vi "Remove Unlogged Channel from Group.vi"(10 "Item Name":string, 11 "References":T1) -> (0 "error out":errorcluster)   [LabVIEW 2015, in "TDMS datalogger editor node.lvclass"]
uses:
  TDMS datalogger editor node.lvclass
  <vilib>/NI/DCAF/Tag Editor Core/Table API/Table Manager/object ref.ctl
  <vilib>/NI/DCAF/Tag Editor Core/Configuration Editor/Classes/Engine Parent/Engine Parent Editor Node.lvclass
  <vilib>/NI/DCAF/Tag Editor Core/Configuration Editor/Classes/Module editor node/module editor node.lvclass
  TDMS datalogger editor node.lvclass/TDMS datalogger editor node.ctl
  <vilib>/NI/DCAF/Tag Editor Core/Table API/Table Manager/Table Manager.lvclass
panel:
  in  "Groups":string(tree)="group1"
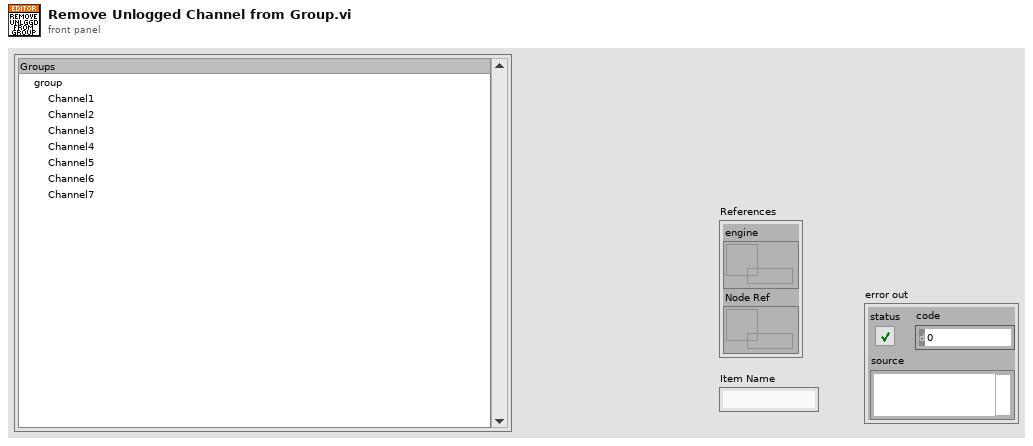
[diagram p1: front panel]
types:
  T1 = typedef "Table Manager.lvlib/Table Manager.lvclass/object ref.ctl" = cluster{"engine":refnum<data-value>, "Node Ref":refnum<data-value>}
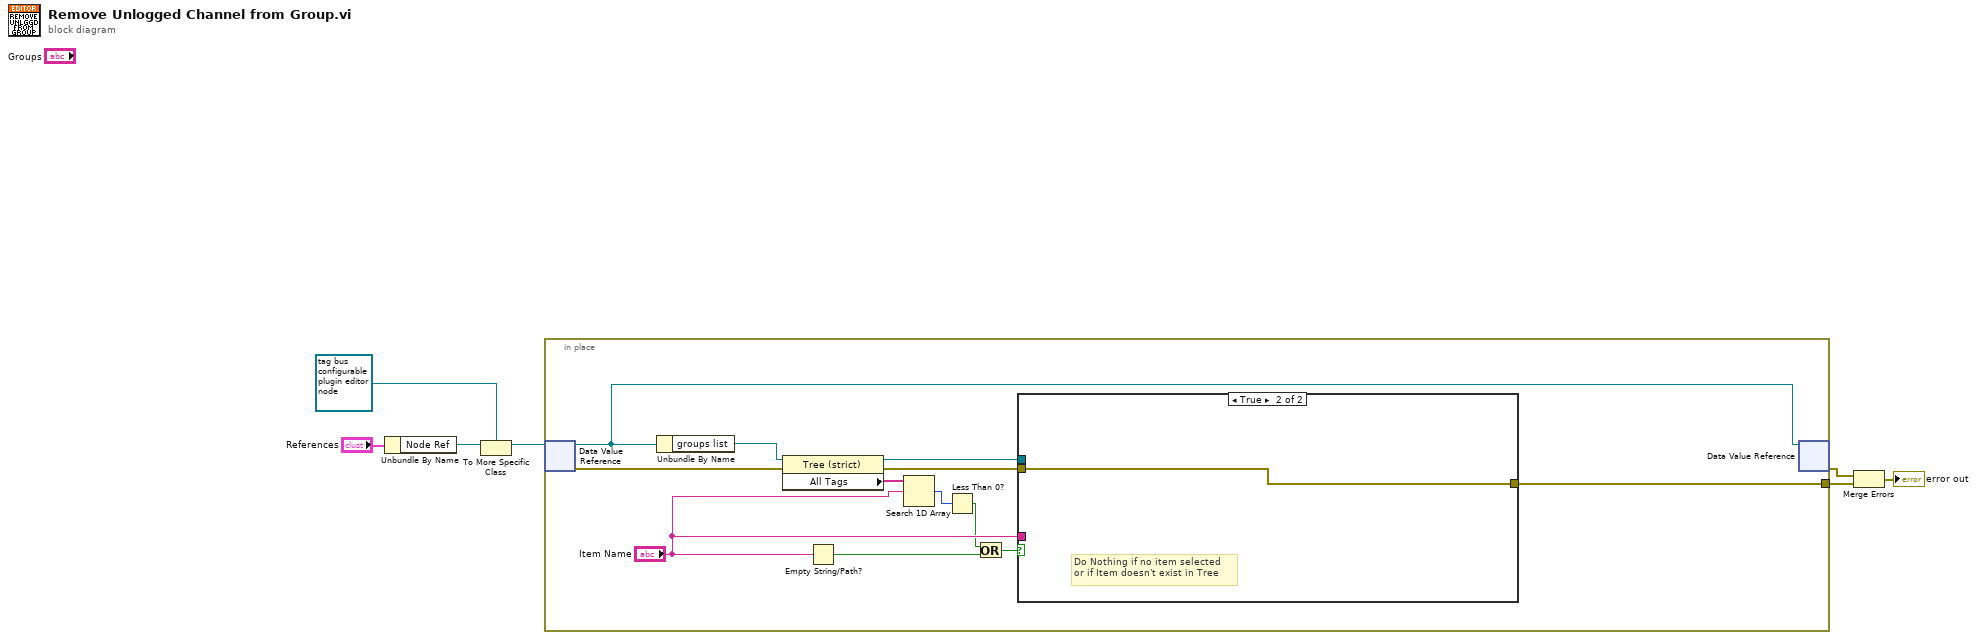
[diagram p0: block diagram]
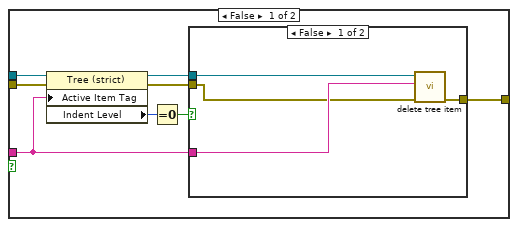
[diagram p2: hidden frame]
diagram:
  n1 = Unbundle By Name("References") -> ("Node Ref"=w4:refnum<data-value>)
  n2 = To More Specific Class(target class=refnum<data-value> refnum ("data value reference"), reference=w4) -> (specific class reference=w2:refnum<data-value>)  [unwired: 1 in, 1 out]
  n3 = in-place {
    in-place-border: [w19] -> w7
    n4 = in-place-dvr #1(w2) -> (w17:refnum<class "TDMS datalogger editor node.lvclass">, w13:errorcluster)
    n5 = Unbundle By Name(w17) -> ("groups list"=w14:refnum<vi>)
    n6 = property class="Tree (strict)"(reference=w14, error in=w13) -> (reference out=w15:refnum<vi>, error out=w16:errorcluster, "All Tags"=w12:string[])
    n7 = Empty String/Path?(string/path="Item Name") -> (empty?=w18:bool)
    n8 = Search 1D Array(1D array=w12, element="Item Name") -> (index of element=w10:i32)  [unwired: 1 in]
    n9 = Less Than 0?(x=w10) -> (x < 0?=w8:bool)
    n10 = Or(x=w8, y=w18) -> (x .or. y?=w9:bool)
    n11 = case shown="True" w9 {
      tunnel: [w27 w33] -> w19
      tunnel: w15 -> [w26 _]
      tunnel: w16 -> [w24 w33]
      tunnel: "Item Name" -> [w20 _]
      frame False {
        n12 = property class="Tree (strict)"(reference=w26, error in=w24, "Active Item Tag"=w20) -> (reference out=w25:refnum<vi>, error out=w23:errorcluster, "Indent Level"=w22:i32)
        n13 = Equal To 0?(x=w22) -> (x = 0?=w21:bool)
        n14 = case shown="False" w21 {
          tunnel: [w31 w32] -> w27
          tunnel: w25 -> [w30 _]
          tunnel: w20 -> [w29 _]
          tunnel: w23 -> [w28 w32]
          frame False {
            n15 = call "delete tree item.vi"("error in"=w28, "Tag"=w29, "tree reference in"=w30) -> ("error out"=w31:errorcluster)  [unwired: 7 in, 1 out]
          }
          frame True {
            # "Do nothing on group items"
          }
        }
      }
      frame True {
        # "Do Nothing if no item selected\nor if Item doesn't exist in Tree"
      }
    }
    n16 = in-place-dvr #1(w17) -> (w6:errorcluster)  [unwired: 1 out]
  }
  n17 = Merge Errors(w6, w7) -> (→"error out":errorcluster)
